vi "Gunsim.vi"() -> ()   [LabVIEW 2015]
uses:
  <vilib>/Utility/file.llb/Write Delimited Spreadsheet (DBL).vi
panel:
  in  "Robot Constants":T1={"Distance from Pivot Point to Drive Mount(in)"=2.0, "Distance from Pivot Point to Arm Mount(in)"=2.0, "Distance from Pivot Point to Launcher(in)"=2.0, "Distance from Pivot Point to Camera(in)"=2.0, "WheelEncoder Ticks/Revolution"=2.0, "Wheel Radius"=2.0, "Triangle Angle(degrees)"=2.0, "Minimum LA Distance(inches)"=2.0, "LA Distance/Tick(inches)"=2.0}
  in  "Other Constants":T2={"Ball Diameter(in)"=10.0, "Air Density(g/in^3)"=0.02, "Drag coefficient"=0.5, "Ball Mass(g)"=300.0, "gravity(in/s^2)"=-386.09, "Minimum Goal Height(in)"=90.0, "Maximum Goal Height(in)"=104.0}
  in  "Sims/angle":i32
  in  "Min Angle":i32
  in  "Max Angle":i32
  in  "Initial Velocity":dbl
  in  "Framerate":i32
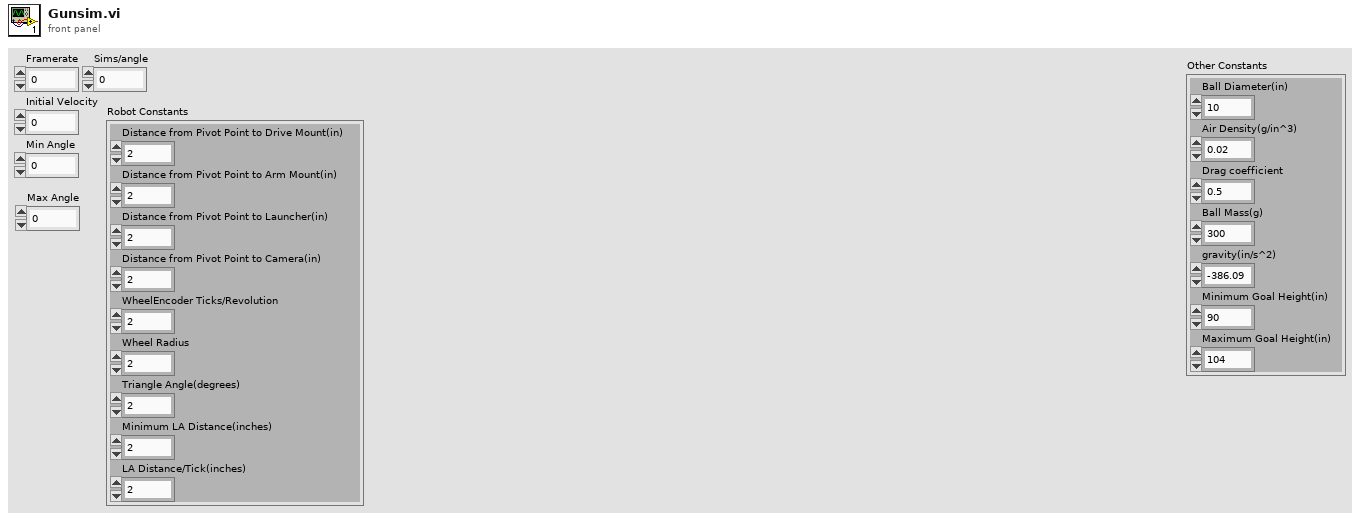
[diagram p1: front panel]
types:
  T1 = cluster{"Distance from Pivot Point to Drive Mount(in)":dbl, "Distance from Pivot Point to Arm Mount(in)":dbl, "Distance from Pivot Point to Launcher(in)":dbl, "Distance from Pivot Point to Camera(in)":dbl, "WheelEncoder Ticks/Revolution":dbl, "Wheel Radius":dbl, "Triangle Angle(degrees)":dbl, "Minimum LA Distance(inches)":dbl, "LA Distance/Tick(inches)":dbl}
  T2 = cluster{"Ball Diameter(in)":dbl, "Air Density(g/in^3)":dbl, "Drag coefficient":dbl, "Ball Mass(g)":dbl, "gravity(in/s^2)":dbl, "Minimum Goal Height(in)":dbl, "Maximum Goal Height(in)":dbl}
  T3 = cluster{"Drag":dbl, "gravity(in/s^2)":dbl, "Minimum Goal Height(in)":dbl, "Maximum Goal Height(in)":dbl, "xspeed":dbl, "yspeed":dbl, "xpos":dbl, "ypos":dbl, "Frametime":dbl, "Output Array":dbl[]}
  T4 = cluster{"Firing Angle":dbl, "Initial Velocity":dbl}
  T5 = cluster{"Minimum Distance":dbl, "Ideal Distance":dbl, "Viable Distances":dbl[], "Maximum Distance":dbl}
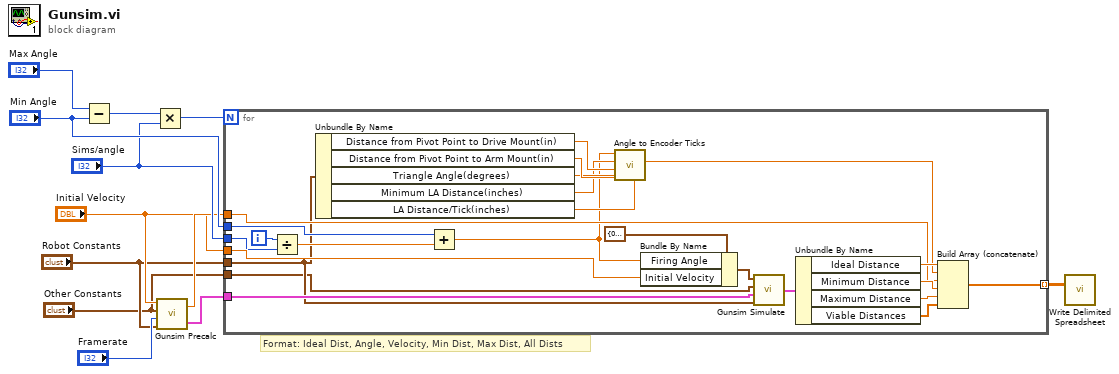
[diagram p0: block diagram]
diagram:
  # "Format: Ideal Dist, Angle, Velocity, Min Dist, Max Dist, All Dists"
  n1 = Subtract(x="Max Angle", y="Min Angle") -> (x-y=w9:i32)
  n2 = Multiply(x=w9, y="Sims/angle") -> (x*y=w8:i32)
  n3 = call "Gunsim Precalc.vi"("Robot Constants"="Robot Constants", "Framerate"="Framerate", "Other Constants"="Other Constants", "Initial Velocity(in/s)"="Initial Velocity") -> ("output cluster"=w5:T3, "Wheel Power(ticks/100ms)"=w4:dbl)
  n4 = for {
    N: w8 -> [_]
    tunnel: "Min Angle" -> [w36]
    tunnel: "Initial Velocity" -> [w28]
    tunnel: [w31] -> w10 mode=indexing
    tunnel: "Sims/angle" -> [w27]
    tunnel: w4 -> [w24]
    tunnel: w5 -> [w22]
    tunnel: "Robot Constants" -> [w21]
    tunnel: "Other Constants" -> [w14]
    i -> [w26]
    n5 = Divide(x=w26, y=w27) -> (x/y=w25:dbl)
    n6 = Unbundle By Name(w21) -> ("Distance from Pivot Point to Drive Mount(in)"=w19:dbl, "Distance from Pivot Point to Arm Mount(in)"=w18:dbl, "Triangle Angle(degrees)"=w17:dbl, "Minimum LA Distance(inches)"=w16:dbl, "LA Distance/Tick(inches)"=w15:dbl)
    n7 = Add(x=w36, y=w25) -> (x+y=w13:dbl)
    n8 = call "Angle to Encoder Ticks.vi"("Length/Rotation"=w15, "Angle between PP and LA at 0(degrees)"=w17, "Distance from PP to Arm Mount(in)"=w18, "Distance from PP to Drive Mount(in)"=w19, "Minimum LA Length(in)"=w16, "Angle(degrees)"=w13) -> ("Rotations"=w20:dbl)  [unwired: 5 in]
    n9 = Bundle By Name(cluster=T4 {"Firing Angle"=0.0, "Initial Velocity"=0.0} ("Parameters"), "Firing Angle"=w13, "Initial Velocity"=w28) -> (w35:T4)
    n10 = call "Gunsim Simulate.vi"("Robot Constants"=w21, "cluster in"=w22, "Other Constants"=w14, "Parameters"=w35) -> ("Range"=w33:T5)
    n11 = Unbundle By Name(w33) -> ("Ideal Distance"=w32:dbl, "Minimum Distance"=w30:dbl, "Maximum Distance"=w29:dbl, "Viable Distances"=w23:dbl[])
    n12 = Build Array (concatenate)(w32, w20, w24, w30, w29, w23) -> (w31:dbl[])
  }
  n13 = call-poly <vilib>:"Write Delimited Spreadsheet.vi"("2D data"=w10) -> ()  [unwired: 13 in, 2 out]
